vi "Output_file_Panel.vi"(0 "Output filename":path=path "/G3_3 HD/Users/Paul/New Disp DB file", 5 "Header":string, 9 "Channel Names":string[](array[string]), 11 "Show panel ?":bool) -> (2 "Cancelled":bool, 3 "Save Full Res Data?":bool, 4 "Output filename Out":path=path "/G3_3 HD/Users/Paul/New Disp DB file", 6 "Header Out":string, 10 "Desired Columns":i32[](array[numeric]), 12 "Summarise mode":T1(ring), 13 "Grouping info":T3[](array[typedef]), 14 "Channels to Tabulate in header Out":i32[](listbox), 15 "Save Plotted rows only?":bool)   [LabVIEW 2020]
uses:
  Controls/Group_Binning.ctl
  Results_plotter_Global.vi
panel:
  in  "Cancel Button":bool
  in  "Channels to Tabulate in header":i32[](listbox)
  in  "Channels to first \"bin\" then output":i32[](listbox)
  in  "Channels to Ouput":i32[](listbox)
  in  "Channel to bin":T2(array[cluster])
  in  "Summarize data":i32(listbox)=2
  in  "OK Button":bool
  in  "Column Selector":i32(listbox)
  in  "Row Selector":i32(listbox)=1
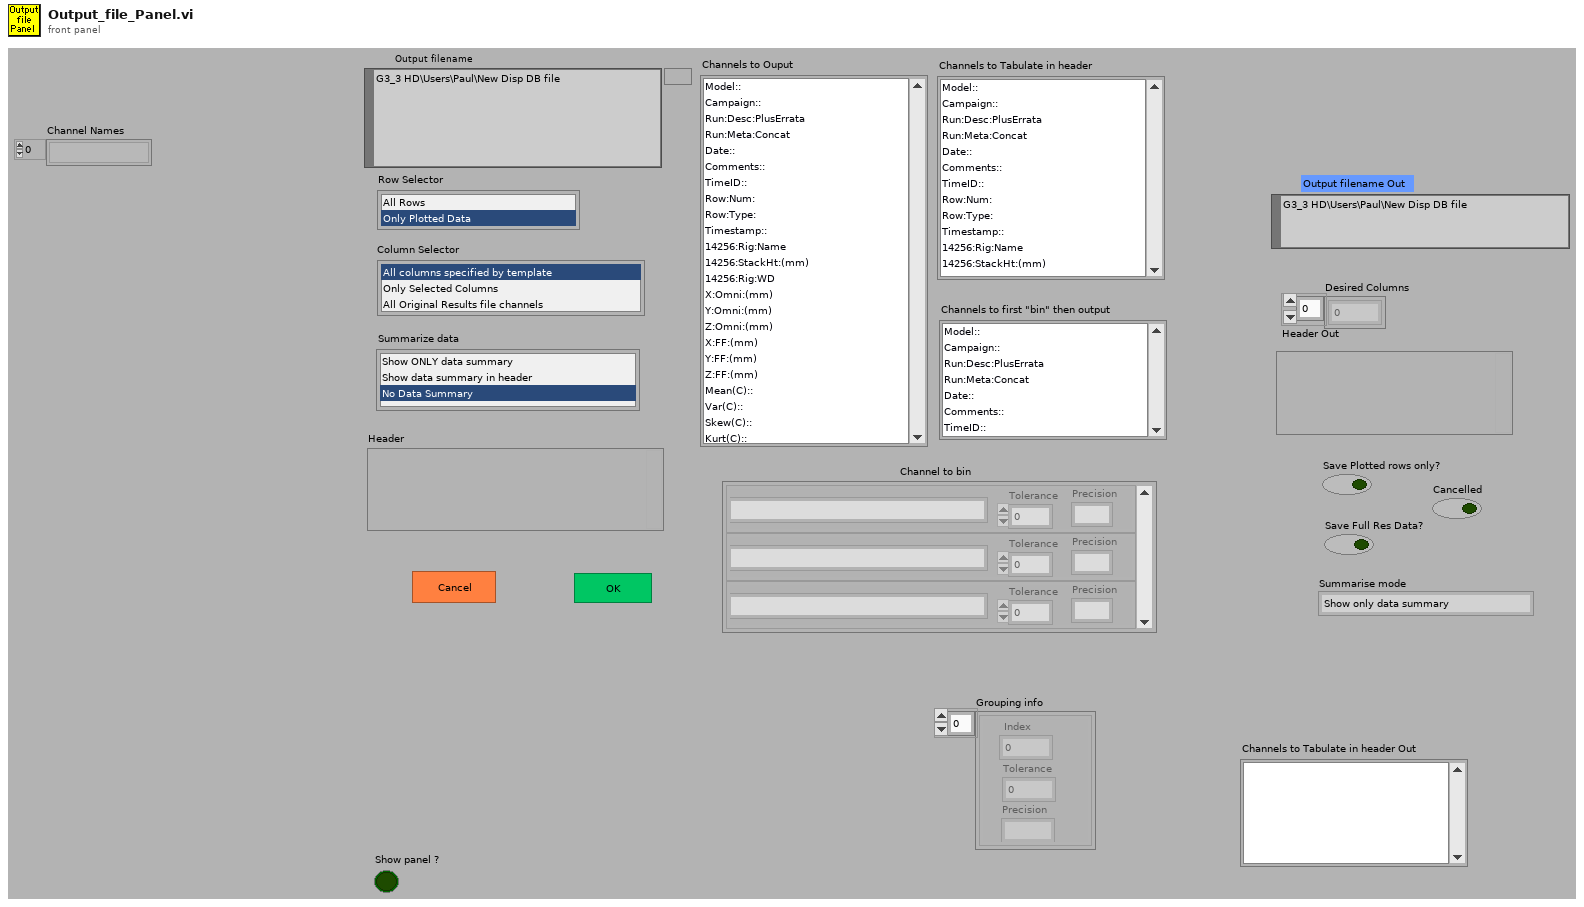
[diagram p1: front panel]
types:
  T1 = enum16{"Show only data summary", "Show data summary", "No data summary"}
  T2 = cluster{"Ch Name":string, "Tolerance":dbl, "Precision":string}[]
  T3 = typedef "Group_Binning.ctl" = cluster{"Index":i32, "Tolerance":dbl, "Precision":string}
  T4 = typedef "Dispose_Channel.ctl" = enum16{"Always", "If Blank", "Never"}
  T5 = cluster{"Ch Name":string, "Tolerance":dbl, "Precision":string}
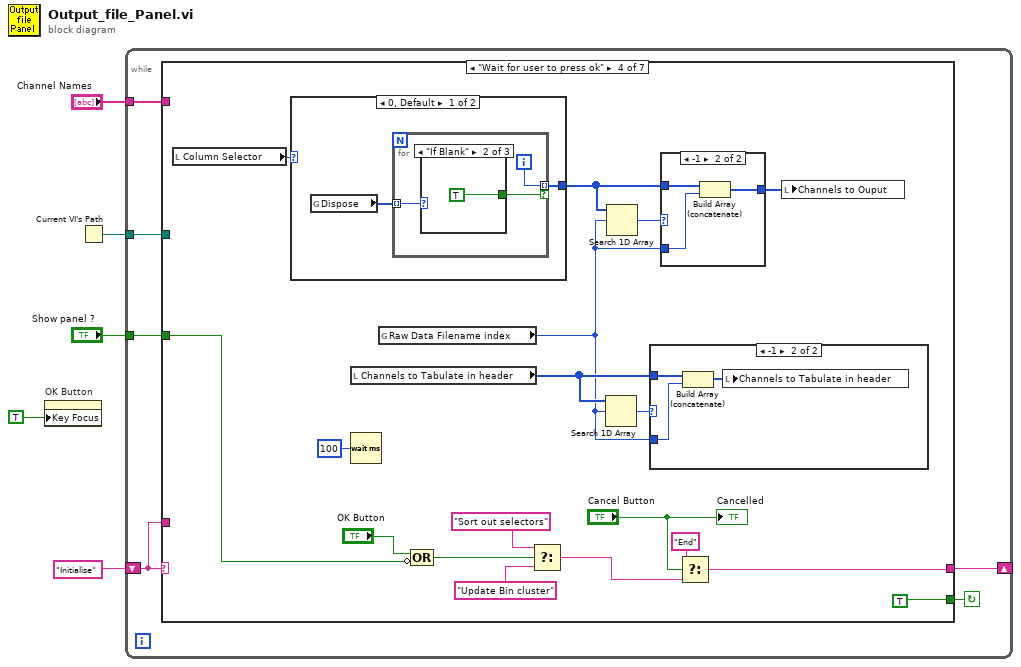
[diagram p0: block diagram]
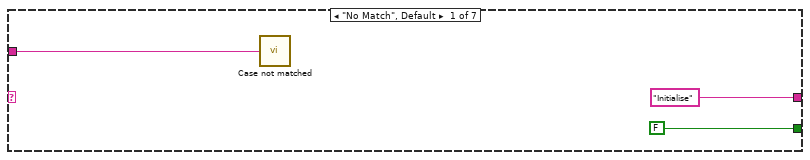
[diagram p2: hidden frame]
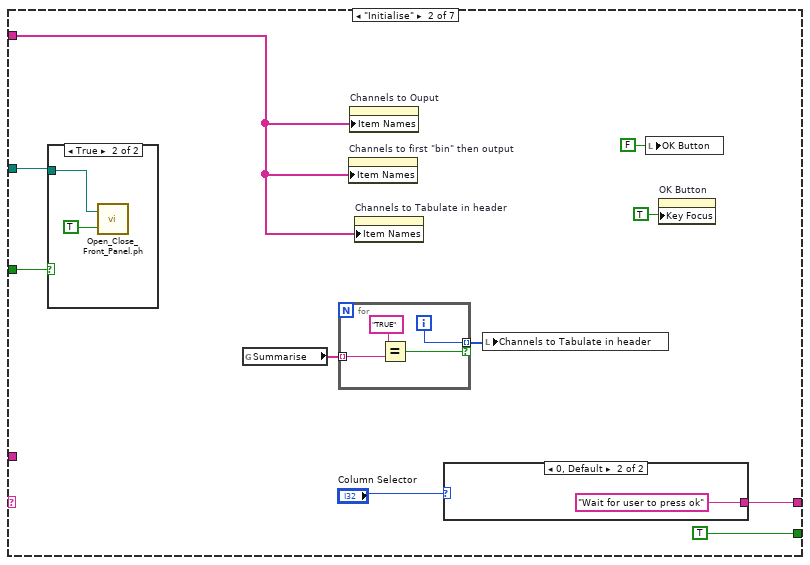
[diagram p3: hidden frame]
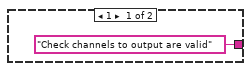
[diagram p4: hidden frame]
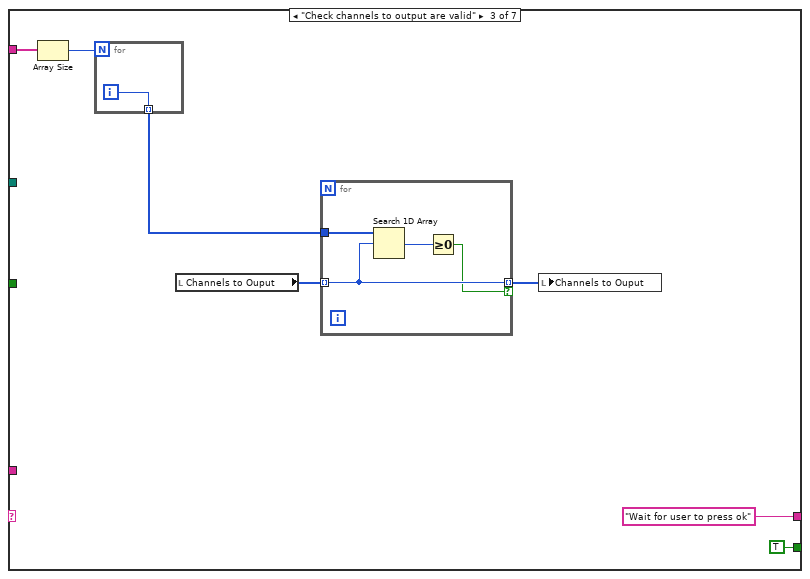
[diagram p6: hidden frame]
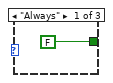
[diagram p9: hidden frame]
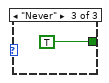
[diagram p10: hidden frame]
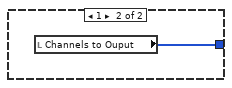
[diagram p11: hidden frame]
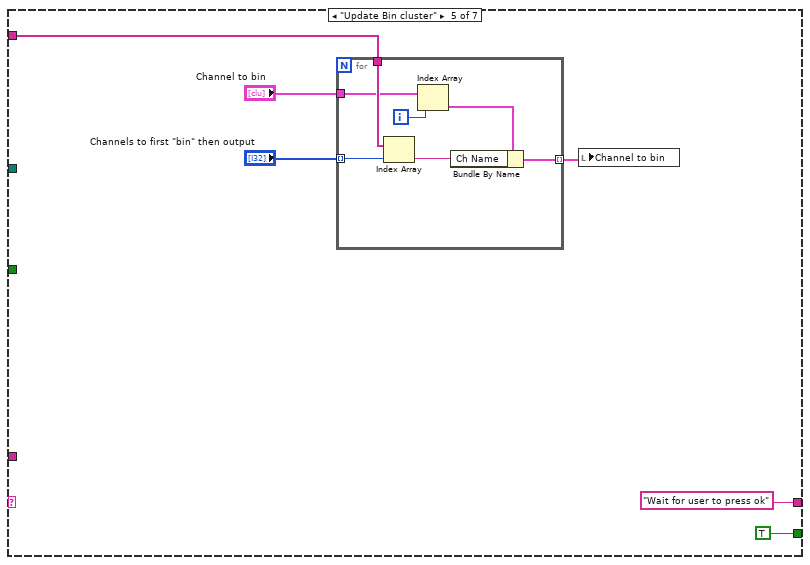
[diagram p12: hidden frame]
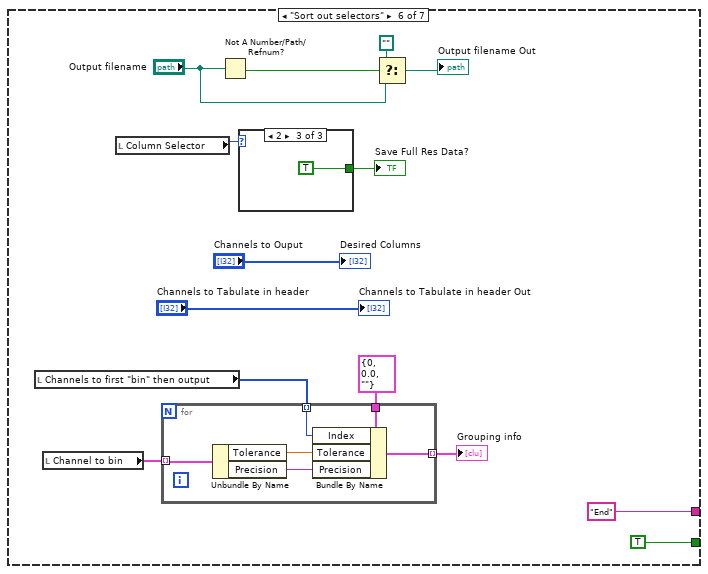
[diagram p13: hidden frame]
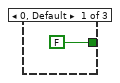
[diagram p14: hidden frame]
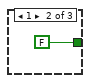
[diagram p15: hidden frame]
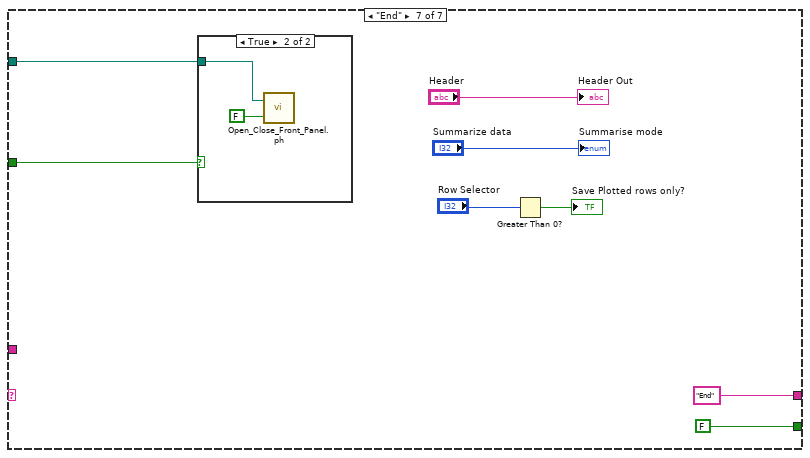
[diagram p16: hidden frame]
diagram:
  n1 = property on="OK Button" class="Bool (strict)"("Key Focus"=TRUE) -> ()  [unwired: 2 in, 2 out]
  n2 = Current VI's Path() -> (path=w3:path)
  n3 = while {
    shift-left: "Initialise" -> [w9]
    shift-right: [w10] -> _
    tunnel: "Show panel ?" -> [w8]
    tunnel: w3 -> [w7]
    tunnel: "Channel Names" -> [w6]
    stop <- w11 continue-if-true
    n4 = case shown="\"Wait for user to press ok\"" w9 {
      tunnel: [FALSE TRUE TRUE TRUE TRUE TRUE FALSE] -> w11
      tunnel: ["Initialise" w24 "Wait for user to press ok" w47 "Wait for user to press ok" "End" ("t") "End"] -> w10
      tunnel: w9 -> [w12 _ _ _ _ _ _]
      tunnel: w8 -> [_ w21 _ w57 _ _ w120]
      tunnel: w7 -> [_ w22 _ _ _ _ w119]
      tunnel: w6 -> [_ w16 w38 _ w81 _ _]
      frame "No Match", Default {
        n5 = call "Case not matched.vi"("Case Name not Matched"=w12) -> ()
      }
      frame "Initialise" {
        n6 = case shown="True" w21 {
          tunnel: w22 -> [_ w28]
          frame False {
          }
          frame True {
            n7 = call "Open_Close_Front_Panel.ph.vi"("Front Panel Window:Open"=TRUE, "VI path"=w28) -> ()  [unwired: 2 out]
          }
        }
        n8 = global read "Results_plotter_Global.vi" "Summarise"() -> (w18:string[])
        n9 = for {
          tunnel: w18 -> [w31] mode=indexing
          tunnel: [w30] -> w17 mode=indexing if=w29
          i -> [w30]
          n10 = Equal?(x="TRUE", y=w31) -> (x = y?=w29:bool)
        }
        n11 = property on="Channels to first \"bin\" then output" class="LstBox (strict)"("Item Names"=w16) -> ()  [unwired: 2 in, 2 out]
        n12 = property on="Channels to Ouput" class="LstBox (strict)"("Item Names"=w16) -> ()  [unwired: 2 in, 2 out]
        n13 = property on="Channels to Tabulate in header" class="LstBox (strict)"("Item Names"=w16) -> ()  [unwired: 2 in, 2 out]
        n14 = case shown="0, Default" "Column Selector" {
          tunnel: ["Check channels to output are valid" "Wait for user to press ok"] -> w24
          frame 1 {
          }
          frame 0, Default {
          }
        }
        n15 = local write "Channels to Tabulate in header"(w17) -> ()
        n16 = local write "OK Button"(FALSE ("OK Button")) -> ()
        n17 = property on="OK Button" class="Bool (strict)"("Key Focus"=TRUE) -> ()  [unwired: 2 in, 2 out]
      }
      frame "Check channels to output are valid" {
        n18 = Array Size(array=w38) -> (size(s)=w39:i32)
        n19 = for {
          N: w39 -> [_]
          tunnel: [w44] -> w36 mode=indexing
          i -> [w44]
        }
        n20 = local read "Channels to Ouput"() -> (w37:i32[])
        n21 = for {
          tunnel: w37 -> [w42] mode=indexing
          tunnel: w36 -> [w43]
          tunnel: [w42] -> w35 mode=indexing if=w40
          n22 = Search 1D Array(1D array=w43, element=w42) -> (index of element=w41:i32)  [unwired: 1 in]
          n23 = Greater Or Equal To 0?(x=w41) -> (x >= 0?=w40:bool)
        }
        n24 = local write "Channels to Ouput"(w35) -> ()
      }
      frame "Wait for user to press ok" {
        n25 = local read "Column Selector"() -> (w51:i32)
        n26 = case shown="0, Default" w51 {
          tunnel: [w70 w78] -> w55
          frame 0, Default {
            n27 = global read "Results_plotter_Global.vi" "Dispose"() -> (w71:T4[])
            n28 = for {
              tunnel: w71 -> [w74] mode=indexing
              tunnel: [w73] -> w70 mode=indexing if=w72
              i -> [w73]
              n29 = case shown="\"If Blank\"" w74 {
                tunnel: [FALSE TRUE TRUE] -> w72
                frame "Always" {
                }
                frame "If Blank" {
                }
                frame "Never" {
                }
              }
            }
          }
          frame 1 {
            n30 = local read "Channels to Ouput"() -> (w78:i32[])
          }
        }
        n31 = local read "Channels to Tabulate in header"() -> (w52:i32[])
        n32 = Wait (ms)(milliseconds to wait=u32 100) -> ()  [unwired: 1 out]
        n33 = global read "Results_plotter_Global.vi" "Raw Data Filename index"() -> (w50:i32)
        n34 = Compound Arithmetic op=OR("OK Button", invert w57) -> (w58:bool)
        n35 = Select(t="Sort out selectors", s=w58, f="Update Bin cluster") -> (s? t:f=w49:string)
        n36 = Search 1D Array(1D array=w52, element=w50) -> (index of element=w53:i32)  [unwired: 1 in]
        n37 = Search 1D Array(1D array=w55, element=w50) -> (index of element=w56:i32)  [unwired: 1 in]
        n38 = case shown="-1" w53 {
          tunnel: w52 -> [_ w65]
          tunnel: w50 -> [_ w64]
          frame Default {
          }
          frame -1 {
            n39 = Build Array (concatenate)(w65, w64) -> (w63:i32[])
            n40 = local write "Channels to Tabulate in header"(w63) -> ()
          }
        }
        n41 = case shown="-1" w56 {
          tunnel: w55 -> [w66 w69]
          tunnel: w50 -> [_ w68]
          tunnel: [w66 w67] -> w54
          frame Default {
          }
          frame -1 {
            n42 = Build Array (concatenate)(w69, w68) -> (w67:i32[])
          }
        }
        n43 = Select(t="End", s="Cancel Button", f=w49) -> (s? t:f=w47:string)
        n44 = local write "Channels to Ouput"(w54) -> ()
        "Cancelled" <- "Cancel Button"
      }
      frame "Update Bin cluster" {
        n45 = for {
          tunnel: "Channels to first \"bin\" then output" -> [w91] mode=indexing
          tunnel: w81 -> [w90]
          tunnel: "Channel to bin" -> [w87]
          tunnel: [w85] -> w79 mode=indexing
          i -> [w88]
          n46 = Index Array(array=w90, index=w91) -> (element=w89:string)
          n47 = Index Array(array=w87, index=w88) -> (element=w86:T5)
          n48 = Bundle By Name(cluster=w86, "Ch Name"=w89) -> (w85:T5)
        }
        n49 = local write "Channel to bin"(w79) -> ()
      }
      frame "Sort out selectors" {
        n50 = local read "Channels to first \"bin\" then output"() -> (w94:i32[])
        n51 = local read "Channel to bin"() -> (w97:T2)
        n52 = local read "Column Selector"() -> (w104:i32)
        n53 = for {
          tunnel: w97 -> [w111] mode=indexing
          tunnel: [w108] -> w96 mode=indexing
          tunnel: w94 -> [w107] mode=indexing
          tunnel: T3 {"Index"=0, "Tolerance"=0.0, "Precision"=""} ("Grouping info") -> [w106]
          n54 = Unbundle By Name(w111) -> ("Tolerance"=w110:dbl, "Precision"=w109:string)
          n55 = Bundle By Name(cluster=w106, "Index"=w107, "Tolerance"=w110, "Precision"=w109) -> (w108:T3)
        }
        "Grouping info" <- w96
        n56 = Not A Number/Path/Refnum?(number/path/refnum="Output filename") -> (NaN/Path/Refnum?=w101:bool)
        n57 = case shown="2" w104 {
          tunnel: [FALSE FALSE TRUE] -> w102
          frame 0, Default {
          }
          frame 1 {
          }
          frame 2 {
          }
        }
        "Save Full Res Data?" <- w102
        n58 = Select(t=path "", s=w101, f="Output filename") -> (s? t:f=→"Output filename Out":path)
        "Desired Columns" <- "Channels to Ouput"
        "Channels to Tabulate in header Out" <- "Channels to Tabulate in header"
      }
      frame "End" {
        n59 = case shown="True" w120 {
          tunnel: w119 -> [_ w124]
          frame False {
          }
          frame True {
            n60 = call "Open_Close_Front_Panel.ph.vi"("Front Panel Window:Open"=FALSE, "VI path"=w124) -> ()  [unwired: 2 out]
          }
        }
        n61 = Greater Than 0?(x="Row Selector") -> (x > 0?=→"Save Plotted rows only?":bool)
        "Header Out" <- "Header"
        "Summarise mode" <- "Summarize data"
      }
    }
  }
